vi "Get Message Class Name.vi"(10 "Message Interface in":refnum<class "Message Interface.lvclass">) -> (2 "Message Interface out":refnum<class "Message Interface.lvclass">)   [LabVIEW 2016, in "Stream Mediator.lvlib" / "Message Interface.lvclass"]
uses:
  <userlib>/Composed Systems/Stream/Mediator/Classes/Message Interface/Message Interface.lvclass
panel:
  out "Class Name":string
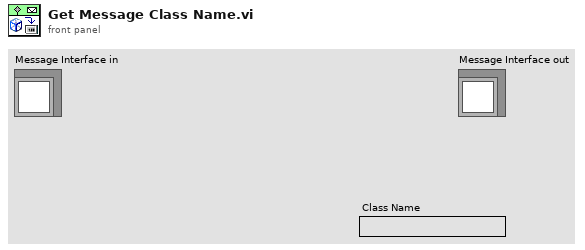
[diagram p1: front panel]
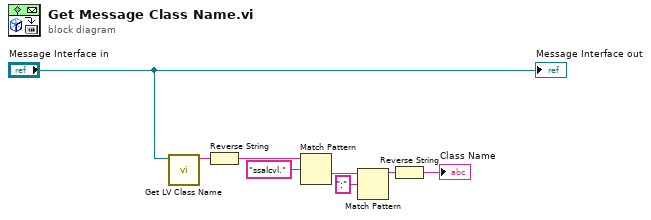
[diagram p0: block diagram]
diagram:
  n1 = call <vilib>:"Get LV Class Name.vi"("object"="Message Interface in") -> ("class name"=w3:string)  [unwired: 9 in, 1 out]
  n2 = Reverse String(1:w3) -> (0:w7:string)
  n3 = Match Pattern(string=w7, regular expression="ssalcvl.") -> (after substring=w4:string)  [unwired: 1 in, 3 out]
  n4 = Match Pattern(string=w4, regular expression=":") -> (before substring=w8:string)  [unwired: 1 in, 3 out]
  n5 = Reverse String(1:w8) -> (0:→"Class Name":string)
  "Message Interface out" <- "Message Interface in"
